vi "Set Origin to (0,0).vi"(8 "error in (no error)":errorcluster, 10 "Save VI (T)":bool=TRUE, 11 "vi path":path) -> (0 "error out":errorcluster)   [LabVIEW 2023]
uses:
  <vilib>/Utility/miscctls.llb/LVPointTypeDef.ctl
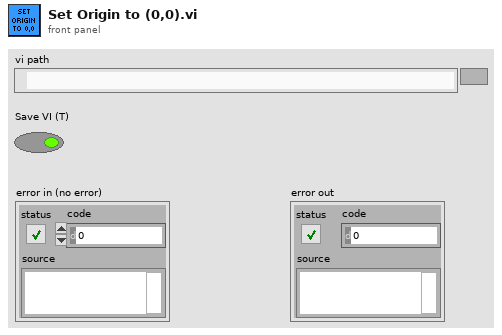
[diagram p1: front panel]
types:
  T1 = typedef "LVPointTypeDef.ctl" = cluster{"Horizontal":i16, "Vertical":i16}
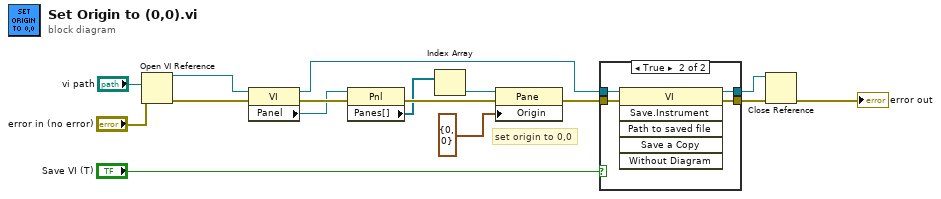
[diagram p0: block diagram]
diagram:
  # "set origin to 0,0"
  n1 = Open VI Reference(vi path="vi path", error in (no error)="error in (no error)") -> (vi reference=w5:refnum<vi>, error out=w3:errorcluster)  [unwired: 4 in]
  n2 = property class="VI"(reference=w5, error in=w3) -> (reference out=w2:refnum<vi>, error out=w15:errorcluster, "Panel"=w4:refnum<vi>)
  n3 = property class="Pnl"(reference=w4, error in=w15) -> (error out=w16:errorcluster, "Panes[]"=w9:refnum<vi>[])  [unwired: 1 out]
  n4 = Index Array(array=w9) -> (element=w8:refnum<vi>)  [unwired: 1 in]
  n5 = property class="Pane"(reference=w8, error in=w16, "Origin"=T1 {"Horizontal"=0, "Vertical"=0} ("Front Panel Window:Minimum Size")) -> (error out=w6:errorcluster)  [unwired: 1 out]
  n6 = case shown="True" "Save VI (T)" {
    tunnel: w6 -> [w18 w22]
    tunnel: [w18 w21] -> w12
    tunnel: [w17 w20] -> w11
    tunnel: w2 -> [w17 w19]
    frame False {
    }
    frame True {
      n7 = invoke class="VI" method="Save.Instrument"(reference=w19, error in=w22) -> (reference out=w20:refnum<vi>, error out=w21:errorcluster)  [unwired: 4 in, 4 out]
    }
  }
  n8 = Close Reference(reference=w11, error in (no error)=w12) -> (error out=→"error out":errorcluster)
